vi "WV_PS_graph.vi"(8 "Power spectrum unit":string(combo), 9 "Time unit":string(combo), 10 "dt":dbl, 11 "Signal in":dbl[](array[numeric])) -> (0 "Power Spectrum / PSD":cluster{"f0":dbl, "df":dbl, "magnitude":dbl[]} {"magnitude" format="%.2p"; "f0" format="%0.2p"; "df" format="%0.2p"}, 3 "output waveform":waveform(dbl))   [LabVIEW 2016]
uses:
  <vilib>/measure/maspectr.llb/FFT Power Spectrum and PSD for 1 Chan.vi
  <vilib>/measure/NI_MAPro.lvlib
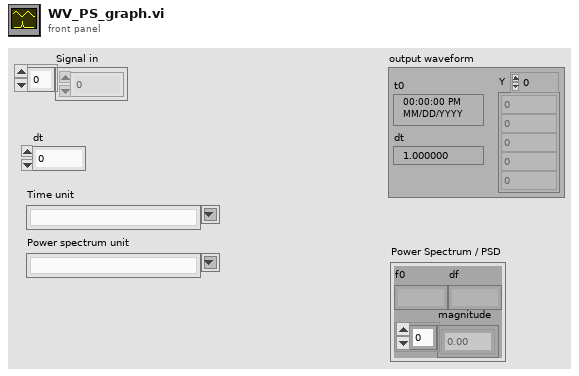
[diagram p1: front panel]
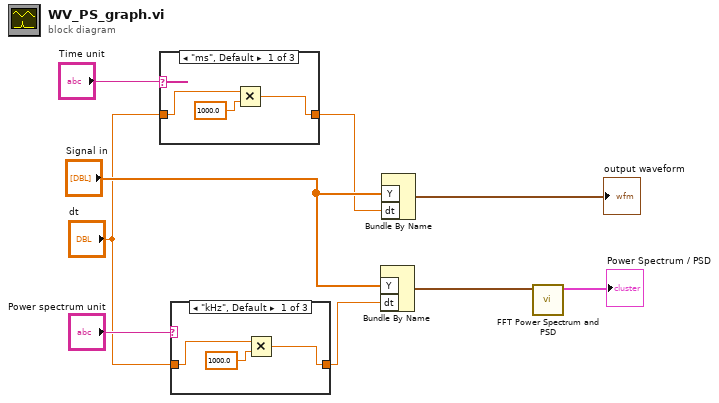
[diagram p0: block diagram]
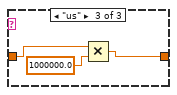
[diagram p3: hidden frame]
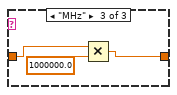
[diagram p5: hidden frame]
diagram:
  n1 = case shown="\"ms\", Default" "Time unit" {
    tunnel: "dt" -> [w12 w13 w16]
    tunnel: [w11 w13 w15] -> w2
    frame "ms", Default {
      n2 = Multiply(x=w12, y=1000.0) -> (x*y=w11:dbl)
    }
    frame "s" {
    }
    frame "us" {
      n3 = Multiply(x=w16, y=1000000.0) -> (x*y=w15:dbl)
    }
  }
  n4 = case shown="\"kHz\", Default" "Power spectrum unit" {
    tunnel: "dt" -> [w19 w20 w23]
    tunnel: [w18 w20 w22] -> w7
    frame "kHz", Default {
      n5 = Multiply(x=w19, y=1000.0) -> (x*y=w18:dbl)
    }
    frame "Hz" {
    }
    frame "MHz" {
      n6 = Multiply(x=w23, y=1000000.0) -> (x*y=w22:dbl)
    }
  }
  n7 = Bundle By Name("Y"="Signal in", "dt"=w7) -> (w6:waveform(dbl))  [unwired: 1 in]
  n8 = Bundle By Name("Y"="Signal in", "dt"=w2) -> (→"output waveform":waveform(dbl))  [unwired: 1 in]
  n9 = call-poly <vilib>:"FFT Power Spectrum and PSD.vi"("time signal"=w6) -> ("Power Spectrum / PSD"=→"Power Spectrum / PSD":cluster{"f0":dbl, "df":dbl, "magnitude":dbl[]})  [unwired: 7 in, 3 out]
